vi "Command builder.vi"(8 "error in":errorcluster, 11 "Config path":path=path "C:/Users/ken_X/Documents/LabVIEW projects/Project-B2/settings/config.xls") -> (0 "error out":errorcluster, 2 "Commands":string[][](array[string]))   [LabVIEW 2021]
uses:
  <vilib>/Utility/file.llb/Read Delimited Spreadsheet (string).vi
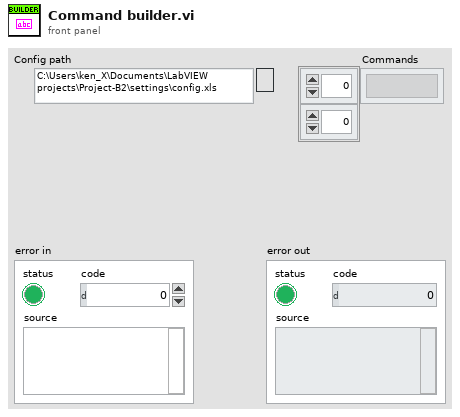
[diagram p1: front panel]
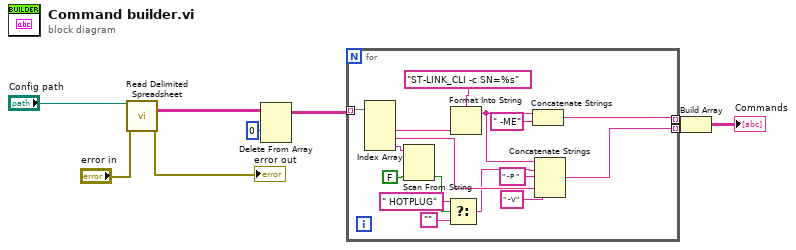
[diagram p0: block diagram]
diagram:
  n1 = call-poly <vilib>:"Read Delimited Spreadsheet.vi"("file path (dialog if empty)"="Config path", "error in (no error)"="error in") -> ("all rows"=w8:string[][], "error out"=→"error out":errorcluster)  [unwired: 8 in, 4 out]
  n2 = Delete From Array(array=w8, index (row)=0) -> (array with subset deleted=w7:string[][])  [unwired: 2 in, 1 out]
  n3 = for {
    tunnel: w7 -> [w25] mode=indexing
    tunnel: [w17] -> w2 mode=indexing
    tunnel: [w16] -> w3 mode=indexing
    n4 = Index Array(array=w25) -> (element #2=w23:string, element #3=w19:string, element #4=w14:string)  [unwired: 4 in, 1 out]
    n5 = Scan From String(input string=w14, default 1=FALSE) -> (output 1=w13:bool)  [unwired: 3 in, 3 out]
    n6 = Select(t=" HOTPLUG", s=w13, f="") -> (s? t:f=w10:string)
    n7 = Format Into String(format string="ST-LINK_CLI -c SN=%s", w23) -> (resulting string=w21:string)  [unwired: 2 in, 1 out]
    n8 = Concatenate Strings(w21, " -ME" ("string")) -> (w16:string)
    n9 = Concatenate Strings(w21, w10, " -P " ("string"), w19, " -V" ("string")) -> (w17:string)
  }
  n10 = Build Array(w3, w2) -> (→"Commands":string[][])
